vi "5p1_HW_Task2_jones6sv.vi"() -> ()   [LabVIEW 2016]
uses:
  <vilib>/express/express arith-compare/Formula/XNode/ExpressFormulaBlockNode.xnode
panel:
  out "Work out":string
  in  "CHR":dbl
  in  "Gender":string(combo)
  in  "Age":dbl
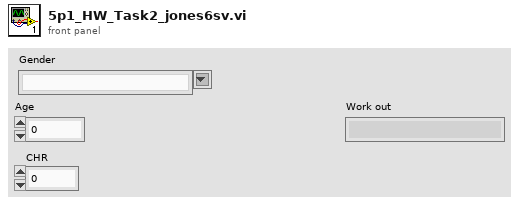
[diagram p1: front panel]
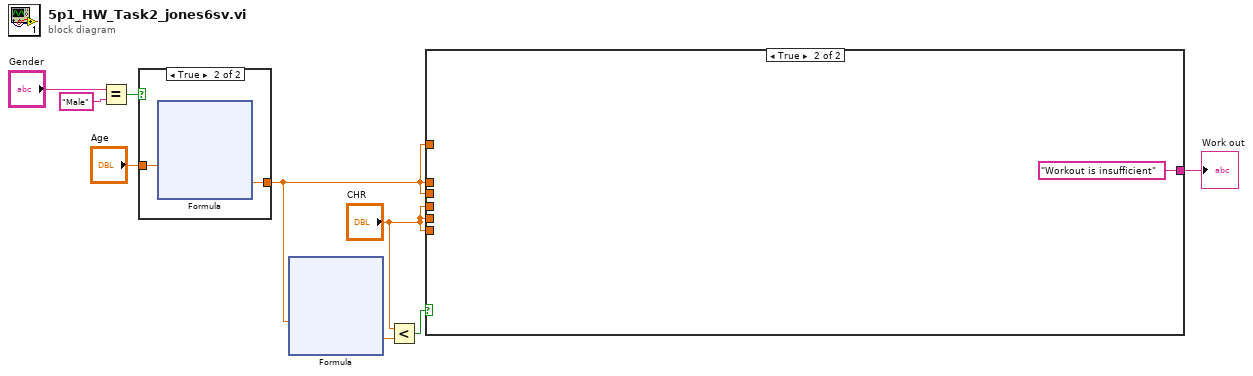
[diagram p0: block diagram]
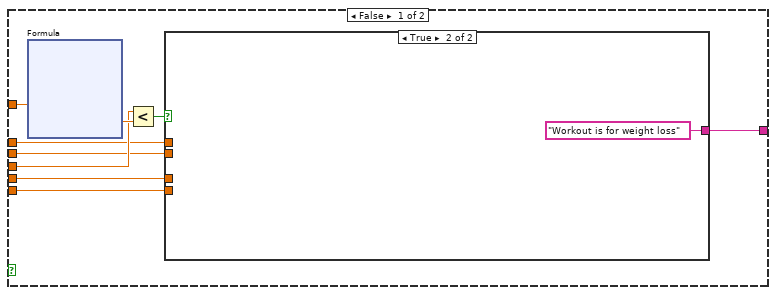
[diagram p2: hidden frame]
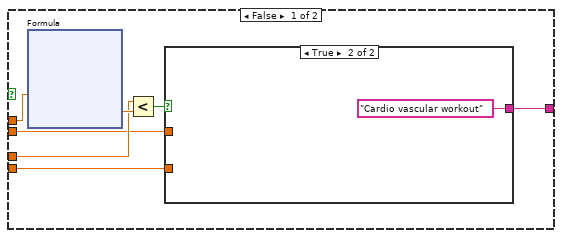
[diagram p3: hidden frame]
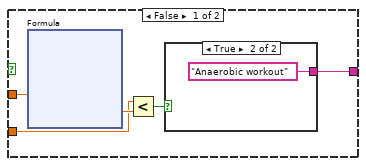
[diagram p4: hidden frame]
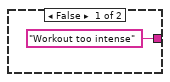
[diagram p5: hidden frame]
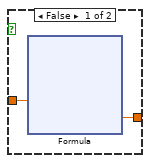
[diagram p6: hidden frame]
diagram:
  n1 = Equal?(x="Gender", y="Male") -> (x = y?=w7:bool)
  n2 = case shown="True" w7 {
    tunnel: "Age" -> [w11 w21]
    tunnel: [w10 w20] -> w3
    frame False {
      n3 = xnode "Formula"("Age"=w11) -> ("Result"=w10:dbl)  [unwired: 1 in, 1 out]
    }
    frame True {
      n4 = xnode "Formula"("Age"=w21) -> ("Result"=w20:dbl)  [unwired: 1 in, 1 out]
    }
  }
  n5 = xnode "Formula"("MHR"=w3) -> ("Result"=w4:dbl)  [unwired: 1 in, 1 out]
  n6 = Less?(x="CHR", y=w4) -> (x < y?=w5:bool)
  n7 = case shown="True" w5 {
    tunnel: w3 -> [w38 _]
    tunnel: "CHR" -> [w36 _]
    tunnel: w3 -> [w34 _]
    tunnel: "CHR" -> [w33 _]
    tunnel: w3 -> [w32 _]
    tunnel: "CHR" -> [w31 _]
    tunnel: [w30 "Workout is insufficient"] -> w1
    frame False {
      n8 = xnode "Formula"("MHR"=w38) -> ("Result"=w37:dbl)  [unwired: 1 in, 1 out]
      n9 = Less?(x=w36, y=w37) -> (x < y?=w35:bool)
      n10 = case shown="True" w35 {
        tunnel: w34 -> [w45 _]
        tunnel: w33 -> [w43 _]
        tunnel: w32 -> [w41 _]
        tunnel: w31 -> [w40 _]
        tunnel: [w39 "Workout is for weight loss"] -> w30
        frame False {
          n11 = xnode "Formula"("MHR"=w45) -> ("Result"=w44:dbl)  [unwired: 1 in, 1 out]
          n12 = Less?(x=w43, y=w44) -> (x < y?=w42:bool)
          n13 = case shown="True" w42 {
            tunnel: w41 -> [w50 _]
            tunnel: w40 -> [w48 _]
            tunnel: [w46 "Cardio vascular workout"] -> w39
            frame False {
              n14 = xnode "Formula"("MHR"=w50) -> ("Result"=w49:dbl)  [unwired: 1 in, 1 out]
              n15 = Less?(x=w48, y=w49) -> (x < y?=w47:bool)
              n16 = case shown="True" w47 {
                tunnel: ["Workout too intense" "Anaerobic workout"] -> w46
                frame False {
                }
                frame True {
                }
              }
            }
            frame True {
            }
          }
        }
        frame True {
        }
      }
    }
    frame True {
    }
  }
  "Work out" <- w1
